vi "Import Mappings.vi"(8 "error in (no error)":errorcluster, 10 "Mapping Path":path, 11 "Loop Data":T1) -> (0 "error out":errorcluster)   [LabVIEW 2016, in "System Mapping Tool.lvlib"]
uses:
  System Mapping Tool.lvlib
  TypeDefs/Loop Data.ctl
  TypeDefs/UI Refs.ctl
  NationalInstruments.VeriStand.SystemDefinitionAPI
  NationalInstruments.VeriStand.SystemStorageUI
  Map Channels (Multiple).vi
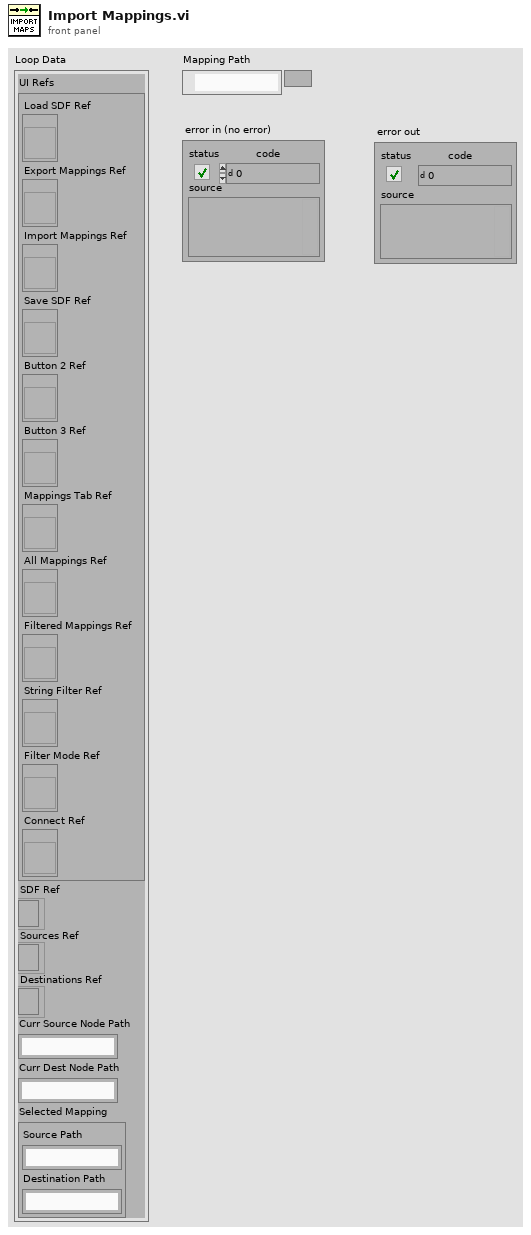
[diagram p1: front panel]
types:
  T1 = typedef "System Mapping Tool.lvlib/Loop Data.ctl" = cluster{"UI Refs":T2, "SDF Ref":refnum<k24>, "Sources Ref":refnum<k24>, "Destinations Ref":refnum<k24>, "Curr Source Node Path":string, "Curr Dest Node Path":string, "Selected Mapping":cluster{"Source Path":string, "Destination Path":string}}
  T2 = typedef "System Mapping Tool.lvlib/UI Refs.ctl" = cluster{"Load SDF Ref":refnum<vi>, "Export Mappings Ref":refnum<vi>, "Import Mappings Ref":refnum<vi>, "Save SDF Ref":refnum<vi>, "Button 2 Ref":refnum<vi>, "Button 3 Ref":refnum<vi>, "Mappings Tab Ref":refnum<vi>, "All Mappings Ref":refnum<vi>, "Filtered Mappings Ref":refnum<vi>, "String Filter Ref":refnum<vi>, "Filter Mode Ref":refnum<vi>, "Connect Ref":refnum<vi>}
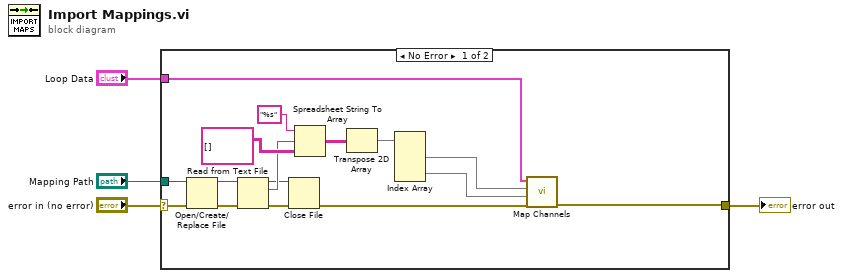
[diagram p0: block diagram]
diagram:
  n1 = case shown="No Error" "error in (no error)" {
    selector: "error in (no error)" -> [w13 w21]
    tunnel: [w5 w21] -> w3
    tunnel: "Mapping Path" -> [w12 _]
    tunnel: "Loop Data" -> [w6 _]
    frame No Error {
      n2 = Open/Create/Replace File(file path (use dialog)=w12, error in=w13) -> (refnum out=w15:refnum<file>, error out=w14:errorcluster)  [unwired: 4 in, 1 out]
      n3 = Read from Text File(file (use dialog)=w15, error in=w14) -> (refnum out=w17:refnum<file>, text=w18:string, error out=w16:errorcluster)  [unwired: 2 in, 1 out]
      n4 = Close File(refnum=w17, error in=w16) -> (error out=w9:errorcluster)  [unwired: 1 out]
      n5 = Spreadsheet String To Array(format string="%s", spreadsheet string=w18, array type (2D Dbl)=string[][] []) -> (array=w11:string[][])  [unwired: 1 in]
      n6 = Transpose 2D Array(2D array=w11) -> (transposed array=w10:string[][])
      n7 = Index Array(array=w10) -> (element #1=w7:string[], element #2=w8:string[])  [unwired: 4 in]
      n8 = call-poly "Map Channels.vi"("error in (no error)"=w9, "Destinations"=w8, "Sources"=w7, "Loop Data"=w6) -> ("error out"=w5:errorcluster)  [unwired: 7 in]
    }
    frame Error {
    }
  }
  "error out" <- w3
